vi "ZCAN_FilterAck.vi"(8 "error in (no error)":errorcluster caption="错误输入（无错误）", 10 "can_index":u32, 11 "can_index_handle":u32) -> (0 "error out":errorcluster caption="错误输出", 2 "can_index(out)":u32, 3 "can_index_handle(out)":u32)   [LabVIEW 2020, in "zlgcan.lvlib"]
uses:
  zlgcan.lvlib
  bin/zlgcan_wrap.dll
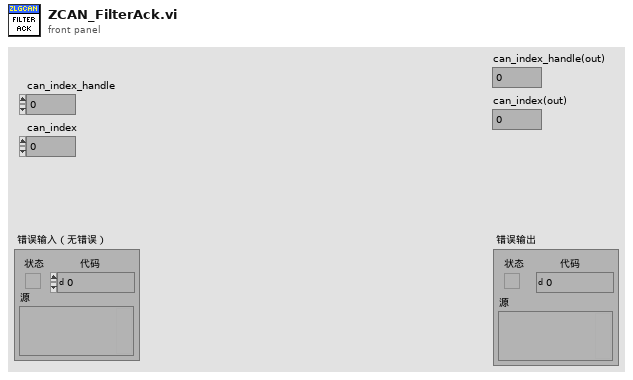
[diagram p1: front panel]
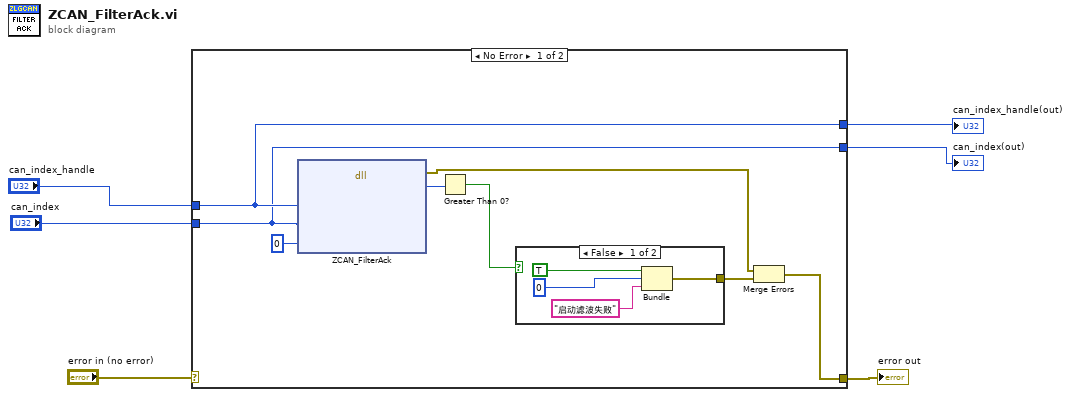
[diagram p0: block diagram]
diagram:
  n1 = case shown="No Error" "error in (no error)" {
    selector: "error in (no error)" -> [_ w19]
    tunnel: [w8 w19] -> w5
    tunnel: "can_index_handle" -> [w12 _]
    tunnel: "can_index" -> [w11 _]
    tunnel: [w12 _] -> w2
    tunnel: [w11 _] -> w1
    frame No Error {
      n2 = dll-call lib="D:/Git/ZLG_USBCANFD/bin/zlgcan_wrap.dll" fn="ZCAN_FilterAck"("device_handle"=w12, "can_index"=w11, "ack"=0 ("clear")) -> (error out=w7:errorcluster, "return"=w10:u32)  [unwired: 6 in, 1 out]
      n3 = Greater Than 0?(x=w10) -> (x > 0?=w9:bool)
      n4 = case shown="False" w9 {
        tunnel: [w15 _] -> w14
        frame False {
          n5 = Bundle("status"=TRUE, "code"=0, "消息"="启动滤波失败") -> (w15:cluster{"status":bool, "code":i32, "消息":string})  [unwired: 1 in]
        }
        frame True {
        }
      }
      n6 = Merge Errors(w7, w14) -> (w8:errorcluster)
    }
    frame Error {
    }
  }
  "error out" <- w5
  "can_index_handle(out)" <- w2
  "can_index(out)" <- w1
